vi "Log_Current_row_to_Execute.vi"(0 "Simulate/Run":T4, 1 "Message":string, 2 "Start of Multi Run Prog":bool, 3 "Traverse line in":T1 {"Row Duration (mins)" format="%#.1f"; "Row No" min=0; "Trace Gas Concentration (%)" min=0.0 format="%#.2f"; "Emission Rate (l/min)" format="%#.2f"; "Tunnel Speed" format="%#.2f"; "Start X" format="%#.2f"; "Start Y" format="%#.2f"; "Start Z" format="%#.2f"; "End X" format="%#.2f"; "End Y" format="%#.2f"; "End Z" format="%#.2f"; "Averaging time (min)" min=0.0 format="%#.2f"}, 4 "Multi Run Log File":path) -> (9 "Traverse line Out":T1 {"Row Duration (mins)" format="%#.1f"; "Row No" min=0; "Trace Gas Concentration (%)" min=0.0 format="%#.2f"; "Emission Rate (l/min)" format="%#.2f"; "Tunnel Speed" format="%#.2f"; "Start X" format="%#.2f"; "Start Y" format="%#.2f"; "Start Z" format="%#.2f"; "End X" format="%#.2f"; "End Y" format="%#.2f"; "End Z" format="%#.2f"; "Averaging time (min)" min=0.0 format="%#.2f"})   [LabVIEW 2010]
uses:
  Traverse_cluster.ctl
  Spacing.ctl
  Controls/Multi_run_mode.ctl
  Controls/User_Specific_mode.ctl
  Controls/Overhead.ctl
  Globals/Trav_pos_global.vi
panel:
  # "X                Y                   Z"
  # "X           Y            Z"
  # "Start"
  # "End"
  # "X           Y            Z"
  # "Start"
  # "End"
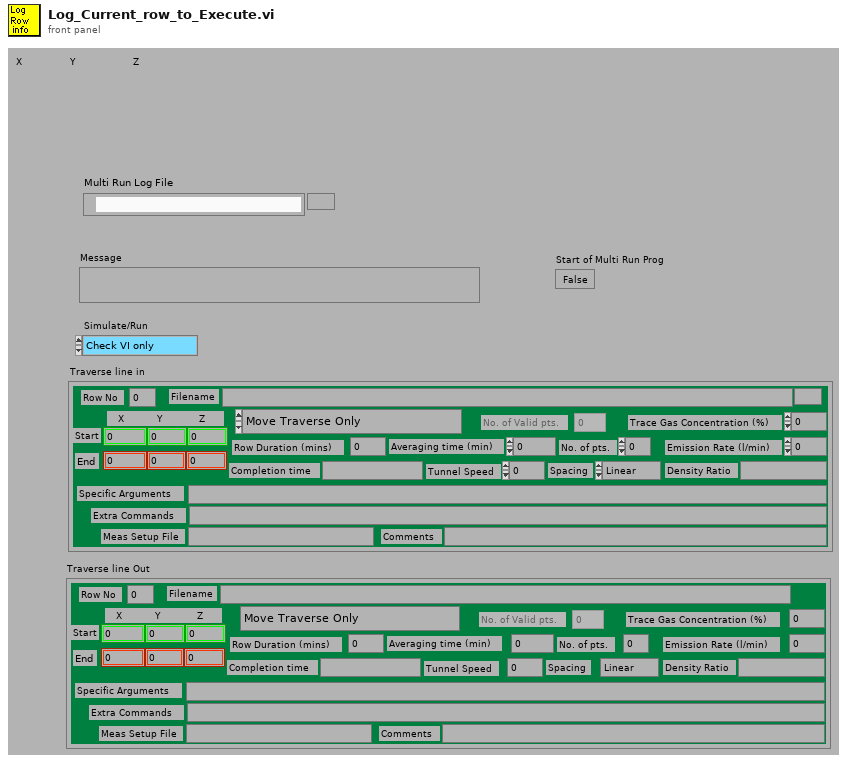
[diagram p1: front panel]
types:
  T1 = typedef "Traverse_cluster.ctl" = cluster{"Start X":dbl, "Start Y":dbl, "Start Z":dbl, "End X":dbl, "End Y":dbl, "End Z":dbl, "No. of pts.":i32, "Spacing":T2, "Filename":path, "Tunnel Speed":dbl, "Averaging time (min)":dbl, "Extra Commands":string, "Specific Arguments":string, "Emission Rate (l/min)":dbl, "Trace Gas Concentration (%)":dbl, "Density Ratio":string, "Comments":string, "Row No":i32, "Row Type Selector":T3, "Completion time":string, "Row Duration (mins)":dbl, "No. of Valid pts.":i32, "Meas Setup File":string}
  T2 = typedef "Spacing.ctl" = enum16{"Linear", "Log", "Gauss", "Specified", "N/A"}
  T3 = typedef "Multi_run_mode.ctl" = enum16{"Move Traverse Only", "Set Tunnel Speed Only", "Set Source Only", "Set Measurement Conditions", "Single Measurement", "Vertical Profile", "Lateral Profile", "Longitudinal Profile", "Explore Volume", "Multi-Axis Profile", "Auto Calibrate", "Meas Fast FID Bkgnd", "Check Beam Power", "Scanning Valve Measurement", "Run VI Named:", "Set ADAM Ch", "Wait (minutes)", "Send Message", "Synchronize With:", "Fall Back to this Row", "Turn Off Row Repeating", "Blank Row"}
  T4 = typedef "User_Specific_mode.ctl" = enum16{"Check VI only", "Run VI"}
  T5 = enum16{"All Channel Names", "Valid Channel Names"}
  T6 = typedef "Overhead.ctl" = enum16{"Update total times", "Read Current Overhead", "Re Scale totals to 3 hrs", "Initialise totals to 3hr"}
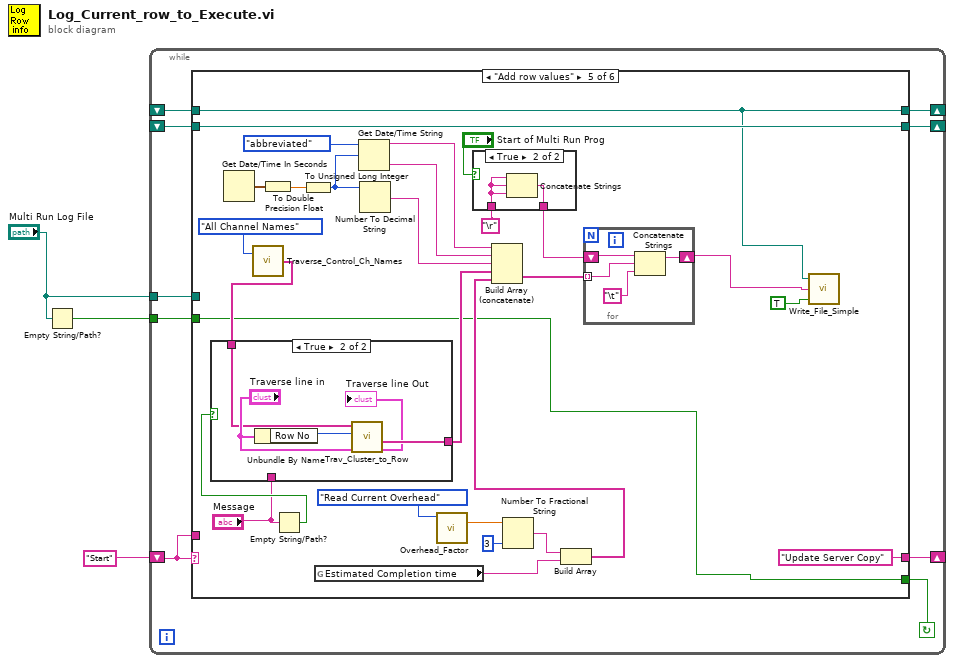
[diagram p0: block diagram]
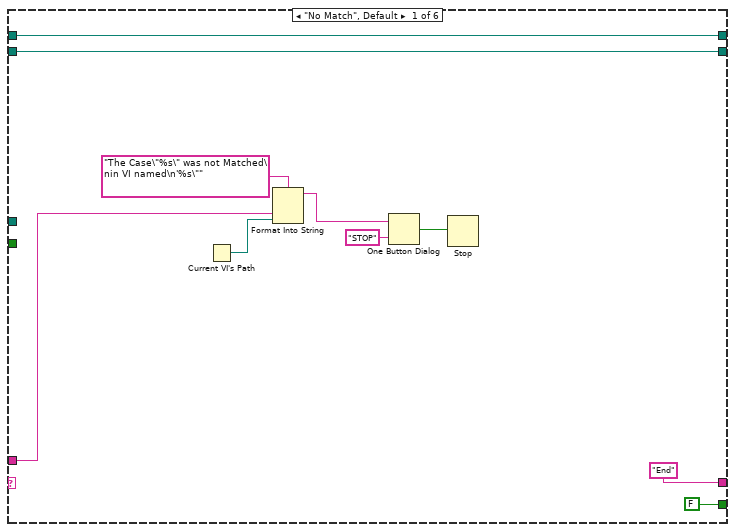
[diagram p2: hidden frame]
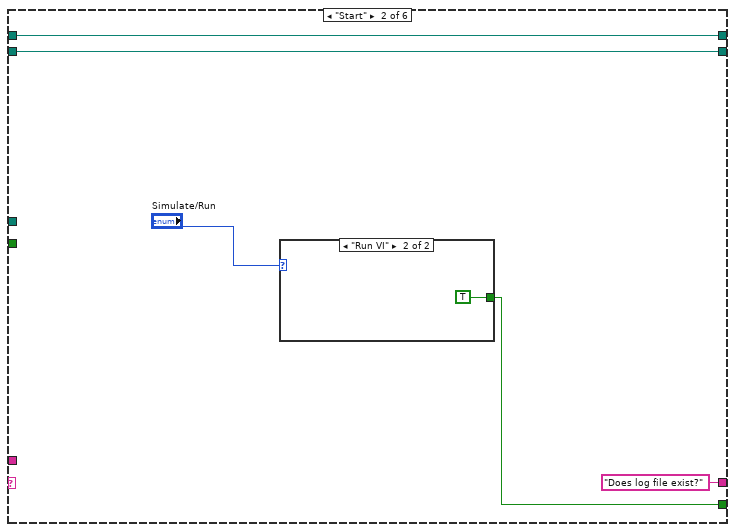
[diagram p3: hidden frame]
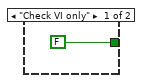
[diagram p4: hidden frame]
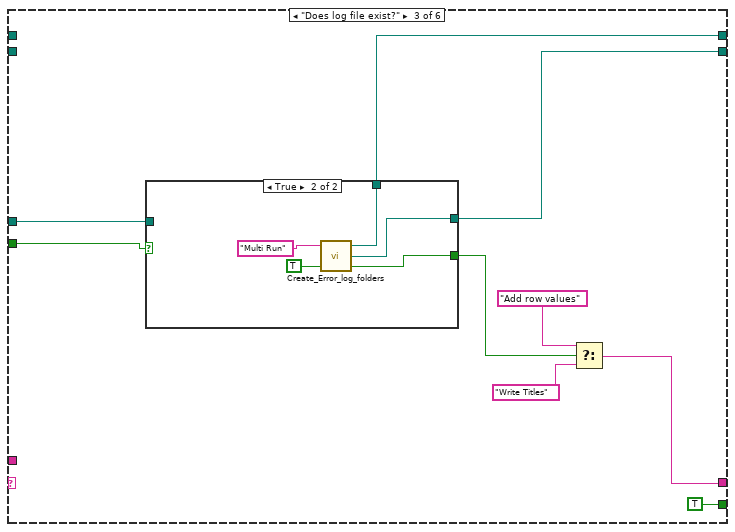
[diagram p5: hidden frame]
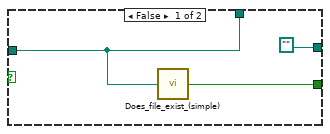
[diagram p6: hidden frame]
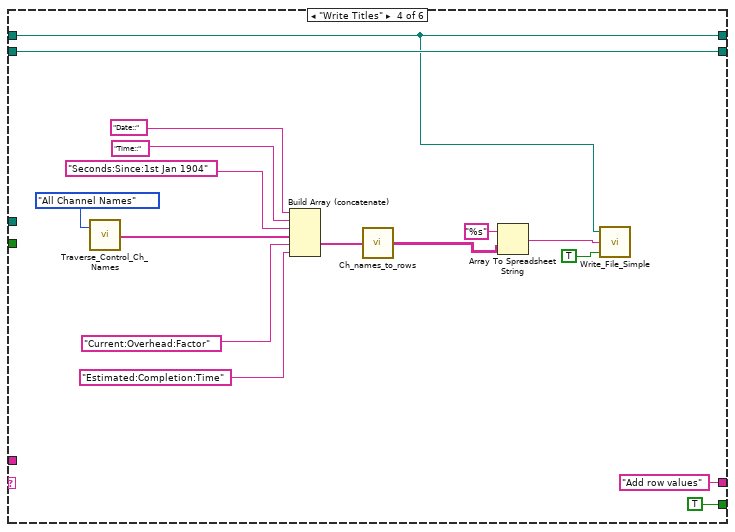
[diagram p7: hidden frame]
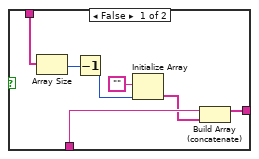
[diagram p9: hidden frame]
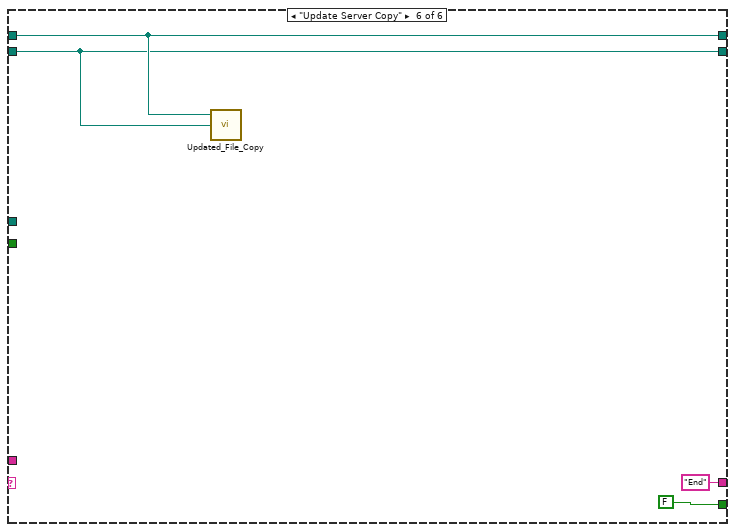
[diagram p10: hidden frame]
diagram:
  n1 = Empty String/Path?(string/path="Multi Run Log File") -> (empty?=w1:bool)
  n2 = while {
    shift-left: _ -> [w9]
    shift-right: [w10] -> _
    shift-left: "Start" -> [w8]
    shift-right: [w11] -> _
    tunnel: "Multi Run Log File" -> [w7]
    tunnel: w1 -> [w6]
    shift-right: [w5] -> _
    shift-left: _ -> [w4]
    stop <- w12 continue-if-true
    n3 = case shown="\"Add row values\"" w8 {
      tunnel: [FALSE ("T button?") w25 TRUE ("T button?") TRUE ("T button?") w67 FALSE] -> w12
      tunnel: ["End" "Does log file exist?" w38 "Add row values" "Update Server Copy" "End" ("f")] -> w11
      tunnel: [w15 w27 w36 w47 w63 w111] -> w10
      tunnel: w9 -> [w15 w27 _ w47 w63 w111]
      tunnel: w8 -> [w14 _ _ _ _ _]
      tunnel: w7 -> [_ _ w32 _ _ _]
      tunnel: w6 -> [_ _ w31 _ w67 _]
      tunnel: [w13 w23 w30 w50 w66 w110] -> w5
      tunnel: w4 -> [w13 w23 _ w50 w66 w110]
      frame "No Match", Default {
        n4 = Current VI's Path() -> (path=w22:path)
        n5 = Format Into String(format string="The Case\"%s\" was not Matched\nin VI named\n'%s\"" ("Format String"), w14, w22) -> (resulting string=w19:string)  [unwired: 2 in, 1 out]
        n6 = One Button Dialog(message=w19, button name ("OK")="STOP") -> (true=w21:bool)
        n7 = Stop(stop? (T)=w21) -> ()
      }
      frame "Start" {
        n8 = case shown="\"Run VI\"" "Simulate/Run" {
          tunnel: [FALSE TRUE] -> w25
          frame "Check VI only" {
          }
          frame "Run VI" {
          }
        }
      }
      frame "Does log file exist?" {
        n9 = case shown="True" w31 {
          tunnel: [w41 w46] -> w36
          tunnel: [w40 w44] -> w35
          tunnel: w32 -> [w41 _]
          tunnel: [path "" w43] -> w30
          frame False {
            n10 = call "Does_file_exist_(simple).vi"("Pathname"=w41) -> ("exists?"=w40:bool)
          }
          frame True {
            n11 = call "Create_Error_log_folders.vi"("Per Day Log File?"=TRUE, "Log Filename"="Multi Run" ("Input Element")) -> ("exists?"=w44:bool, "Server copy Location"=w43:path, "Local Log File"=w46:path)  [unwired: 1 in]
          }
        }
        n12 = Select(t="Add row values", s=w35, f="Write Titles") -> (s? t:f=w38:string)
      }
      frame "Write Titles" {
        n13 = call "Traverse_Control_Ch_Names.vi"("Mode"=T5."All Channel Names") -> ("Channel names"=w56:string[])  [unwired: 1 in]
        n14 = Build Array (concatenate)("Date::", "Time::", "Seconds:Since:1st Jan 1904", w56, "Current:Overhead:Factor", "Estimated:Completion:Time") -> (w53:string[])
        n15 = call "Ch_names_to_rows.vi"("Channel Names"=w53) -> ("3 Row names"=w52:string[][])
        n16 = Array To Spreadsheet String(array=w52, 3:"%s" ("format string")) -> (spreadsheet string=w48:string)  [unwired: 1 out]
        n17 = call "Write_File_Simple.vi"("append to file? (new file:F)"=TRUE, "character string"=w48, "file path"=w47) -> ()  [unwired: 2 out]
      }
      frame "Add row values" {
        n18 = Get Date/Time In Seconds() -> (seconds since 1Jan1904=w68:timestamp)
        n19 = call "Traverse_Control_Ch_Names.vi"("Mode"=T5."All Channel Names") -> ("Channel names"=w80:string[])  [unwired: 1 in]
        n20 = To Double Precision Float(number=w68) -> (double precision float=w89:dbl)
        n21 = Empty String/Path?(string/path="Message") -> (empty?=w82:bool)
        n22 = case shown="True" w82 {
          tunnel: w80 -> [w99 w103]
          tunnel: [w97 w102] -> w84
          tunnel: "Message" -> [w100 _]
          frame False {
            n23 = Array Size(array=w99) -> (size(s)=w96:i32)
            n24 = Decrement(x=w96) -> (x-1=w95:i32)
            n25 = Initialize Array("", w95) -> (w94:string[])
            n26 = Build Array (concatenate)(w100, w94) -> (w97:string[])
          }
          frame True {
            n27 = Unbundle By Name("Traverse line in") -> ("Row No"=w105:i32)
            n28 = call "Trav_Cluster_to_Row.vi"("Traverse line in"="Traverse line in", "Row Number"=w105, "Channel names"=w103) -> ("Traverse line Out"=→"Traverse line Out":T1, "Channel Values Out"=w102:string[])  [unwired: 3 out]
          }
        }
        n29 = To Unsigned Long Integer(number=w89) -> (unsigned 32bit integer=w90:u32)
        n30 = global read "Trav_pos_global.vi" "Estimated Completion time"() -> (w77:string)
        n31 = Get Date/Time String(date format (0)=enum16{"short", "long", "abbreviated"}."abbreviated", seconds (now)=w90) -> (date string=w88:string, time string=w87:string)  [unwired: 1 out]
        n32 = Number To Decimal String(number=w90) -> (decimal integer string=w86:string)  [unwired: 1 out]
        n33 = call "Overhead_Factor.vi"("Mode"=Overhead."Read Current Overhead") -> ("Current Overhead Factor"=w70:dbl)  [unwired: 3 in]
        n34 = case shown="True" "Start of Multi Run Prog" {
          tunnel: [w91 w93] -> w73
          tunnel: "\r" -> [w91 w92]
          frame False {
          }
          frame True {
            n35 = Concatenate Strings(w92, w92, w92) -> (w93:string)
          }
        }
        n36 = Number To Fractional String(number=w70, precision (6)=i16 3) -> (F-format string=w78:string)  [unwired: 2 out]
        n37 = Build Array(w78, w77) -> (w76:string[])
        n38 = Build Array (concatenate)(w88, w87, w86, w84, w76) -> (w85:string[])
        n39 = for {
          shift-right: [w108] -> w64
          shift-left: w73 -> [w109]
          tunnel: w85 -> [w107] mode=indexing
          n40 = Concatenate Strings(w109, w107, "\t") -> (w108:string)
        }
        n41 = call "Write_File_Simple.vi"("append to file? (new file:F)"=TRUE, "character string"=w64, "file path"=w63) -> ()  [unwired: 2 out]
      }
      frame "Update Server Copy" {
        n42 = call "Updated_File_Copy.vi"("Target Path"=w110, "Source Path"=w111) -> ()  [unwired: 2 out]
      }
    }
  }
